vi "Shutdown.vi"(8 "error in (no error)":errorcluster, 11 "SLSC Switch Consumer in":refnum<class "SLSC Switch Consumer.lvclass">=refnum) -> (0 "error out":errorcluster, 3 "SLSC Switch Consumer out":refnum<class "SLSC Switch Consumer.lvclass">)   [LabVIEW 2017, in "SLSC Switch Messaging.lvlib" / "SLSC Switch Consumer.lvclass"]
uses:
  SLSC Switch Consumer.lvclass
  <vilib>/SLSC_Switch/SLSC Switch.lvlib
  <vilib>/userdefined/High Color/SLSC_Switch/nislscslSession.ctl
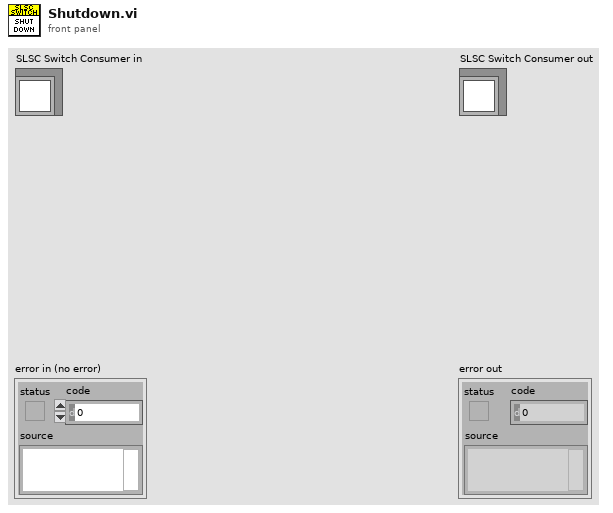
[diagram p1: front panel]
types:
  T1 = typedef "nislscslSession.ctl" = refnum<k20>
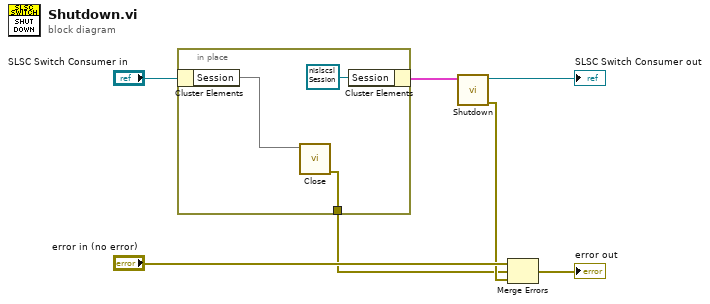
[diagram p0: block diagram]
diagram:
  n1 = in-place {
    in-place-border: [w10] -> w1
    n2 = in-place-cluster #1("SLSC Switch Consumer in") -> ("Session"=w9)
    n3 = call <vilib>:"Close.vi"("session in"=w9) -> ("error out"=w10:errorcluster)  [unwired: 10 in]
    n4 = in-place-cluster #1("Session"=T1 refnum) -> (w2:cluster{})
  }
  n5 = call-parent "Shutdown.vi"("Abstract Consumer in"=w2) -> ("error out"=w5:errorcluster, "Abstract Consumer out"=→"SLSC Switch Consumer out":refnum<class "SLSC Switch Consumer.lvclass">)  [unwired: 9 in]
  n6 = Merge Errors("error in (no error)", w1, w5) -> (→"error out":errorcluster)
